vi "PH Hamming Distance.vi"(10 "Hash B":u64 format="%x", 11 "Hash A":u64 format="%x") -> (3 "Hamming Distance":i32)   [LabVIEW 2014, in "Perceptual Hash Comparison.lvclass"]
uses:
  Perceptual Hash Comparison.lvclass
  Perceptual Hash Comparison/phash DLL/pHash.dll
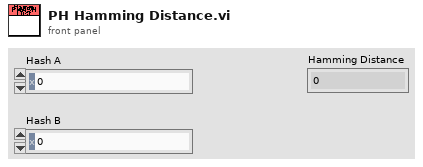
[diagram p1: front panel]
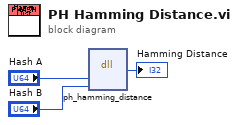
[diagram p0: block diagram]
diagram:
  n1 = dll-call lib="D:/Code/LabVIEW Reddit Coding Challenge - June 2021/Perceptual Hash Comparison/phash DLL/pHash.dll" fn="ph_hamming_distance"("hasha"="Hash A", "hashb"="Hash B") -> ("return type"=→"Hamming Distance":i32)  [unwired: 5 in, 2 out]
